vi "Read magnet system configuration.vi"(8 "error in (no error)":errorcluster, 11 "MAG config file path":path) -> (0 "error out":errorcluster, 3 "Magnet Constantsout":T1={"Switch resistant [K]"=5.0, "Switch superconducting [K]"=4.0, "First stage critical temperature [K]"=50.0, "Second stage critical temperature [K]"=5.0, "Inner magnet critical temperature [K]"=6.0, "Outer magnet critical temperature [K]"=5.0, "Field Constant [T/A]"=0.14911, "Maximum Current [A]"=107.3, "Maximum field [T]"=16.0, "Maximum source ramp [A/s]"=0.5, "Source precision [T]"=2e-05, "Ramp limits [A/s]"=[0.0506, 0.038, 0.0285, 0.0213, 0.0104], "Field limits [T]"=[3.0, 9.6, 13.3, 15.5, 16.0], "SMS"="COM3", "LSC218"="COM1"})   [LabVIEW 2017, in "Magnet module.lvlib"]
doc: "Reads an INI file with magnet configuration data, for example port names and maximum ramp/field constants.\nConsiderable build-in function: searching for SMS serial port"
uses:
  Magnet module.lvlib
  ctl/Magnet config constants.ctl
  <vilib>/Utility/config.llb/NI_LVConfig.lvlib
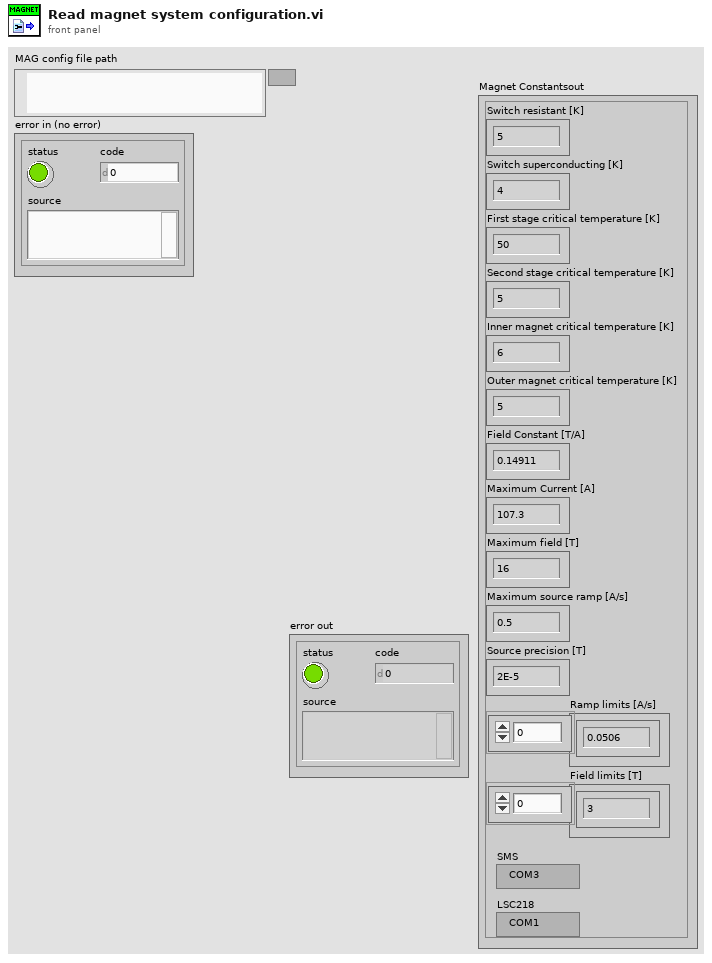
[diagram p1: front panel]
types:
  T1 = typedef "Magnet module.lvlib/Magnet config constants.ctl" = cluster{"Switch resistant [K]":dbl, "Switch superconducting [K]":dbl, "First stage critical temperature [K]":dbl, "Second stage critical temperature [K]":dbl, "Inner magnet critical temperature [K]":dbl, "Outer magnet critical temperature [K]":dbl, "Field Constant [T/A]":dbl, "Maximum Current [A]":dbl, "Maximum field [T]":dbl, "Maximum source ramp [A/s]":dbl, "Source precision [T]":dbl, "Ramp limits [A/s]":dbl[], "Field limits [T]":dbl[], "SMS":refnum<visa-resource-name>, "LSC218":refnum<visa-resource-name>}
  T2 = typedef "NI_LVConfig.lvlib/Config Data RefNum.ctl" = refnum<k1>
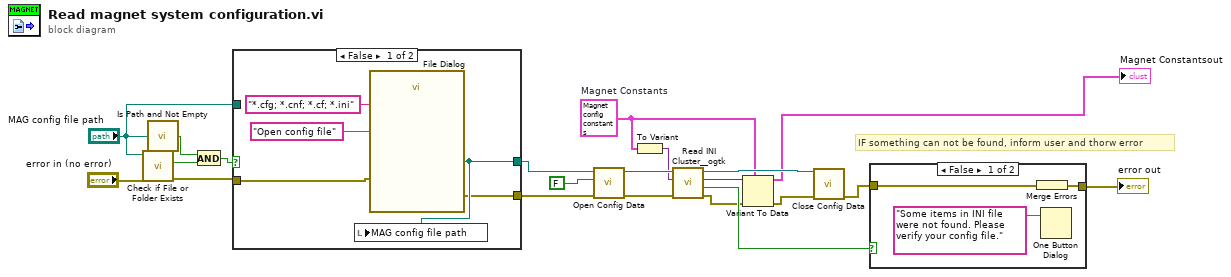
[diagram p0: block diagram]
diagram:
  w2 = T1 {"Switch resistant [K]"=5.0, "Switch superconducting [K]"=4.0, "First stage critical temperature [K]"=50.0, "Second stage critical temperature [K]"=5.0, "Inner magnet critical temperature [K]"=6.0, "Outer magnet critical temperature [K]"=5.0, "Field Constant [T/A]"=0.14911, "Maximum Current [A]"=107.3, "Maximum field [T]"=16.0, "Maximum source ramp [A/s]"=0.5, "Source precision [T]"=2e-05, "Ramp limits [A/s]"=[0.0506, 0.038, 0.0285, 0.0213, 0.0104], "Field limits [T]"=[3.0, 9.6, 13.3, 15.5, 16.0], "SMS"="COM3", "LSC218"="COM1"}  # Magnet Constants
  # "IF something can not be found, inform user and thorw error"
  n1 = call <vilib>:"Check if File or Folder Exists.vi"("error in (no error)"="error in (no error)", "path"="MAG config file path") -> ("error out"=w10:errorcluster, "file or folder exists?"=w7:bool)  [unwired: 7 in, 1 out]
  n2 = call <vilib>:"Is Path and Not Empty.vi"("path"="MAG config file path") -> ("Is Path and Not Empty?"=w5:bool)  [unwired: 4 in]
  n3 = And(x=w5, y=w7) -> (x .and. y?=w6:bool)
  n4 = case shown="False" w6 {
    tunnel: [w24 w28] -> w13
    tunnel: "MAG config file path" -> [_ w28]
    tunnel: [w23 w27] -> w12
    tunnel: w10 -> [w22 w27]
    frame False {
      n5 = call "File Dialog"("prompt"="Open config file" ("default name"), "error in"=w22, "pattern (all files)"="*.cfg; *.cnf; *.cf; *.ini") -> ("selected path"=w24:path, "error out"=w23:errorcluster)  [unwired: 9 in, 2 out]
      n6 = local write "MAG config file path"(w24) -> ()
    }
    frame True {
    }
  }
  n7 = call <vilib>:"Open Config Data.vi"("error in (no error)"=w12, "create file if necessary (T)"=FALSE, "configuration file path"=w13) -> ("error out"=w8:errorcluster, "refnum"=w9:T2)  [unwired: 6 in, 1 out]
  n8 = To Variant(anything=w2) -> (Variant=w1:variant)
  n9 = call <userlib>:"Read INI Cluster__ogtk.vi"("error in (no error)"=w8, "INI Fomatted Cluster Type"=w1, "refnum"=w9) -> ("error out"=w15:errorcluster, "all found?"=w19:bool, "INI Fomatted Cluster"=w20:variant, "dup refnum"=w18:T2)  [unwired: 4 in, 1 out]
  n10 = Variant To Data(error in=w15, type=w2, Variant=w20) -> (data=→"Magnet Constantsout":T1, error out=w14:errorcluster)
  n11 = call <vilib>:"Close Config Data.vi"("error in (no error)"=w14, "refnum"=w18) -> ("error out"=w17:errorcluster)  [unwired: 8 in, 1 out]
  n12 = case shown="False" w19 {
    tunnel: [w29 w32] -> w16
    tunnel: w17 -> [w30 w32]
    frame False {
      n13 = Merge Errors(w30) -> (w29:errorcluster)
      n14 = One Button Dialog(message="Some items in INI file were not found. Please verify your config file.") -> ()  [unwired: 1 in, 1 out]
    }
    frame True {
    }
  }
  "error out" <- w16
